vi "Event Log Monitor.vi"(8 "error in":errorcluster) -> (0 "error out":errorcluster, 3 "Log File Refnum":refnum<file>)   [LabVIEW 2019]
doc: "Does 2 Functions\n\n1. Creates log file name with date/time stamp upon first run\n2. Monitors log file size and closes current file and creates a new one when size limit is reached."
uses:
  Globals and Definitions/Initialization Globals.vi
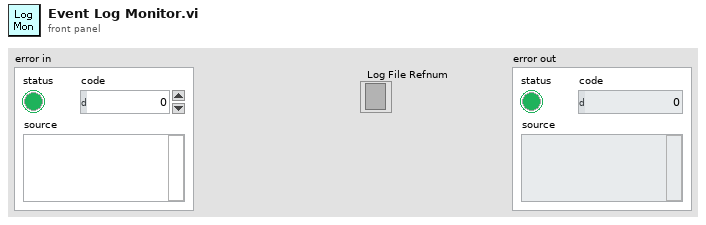
[diagram p1: front panel]
types:
  T1 = enum16{"open", "replace", "create", "open or create", "replace or create", "replace or create with confirmation"}
  T2 = typedef "LVDateTimeRec.ctl" = cluster{"fractional second":dbl, "second":i32, "minute":i32, "hour":i32, "day of month":i32, "month":i32, "year":i32, "day of week":i32, "day of year":i32, "DST":i32}
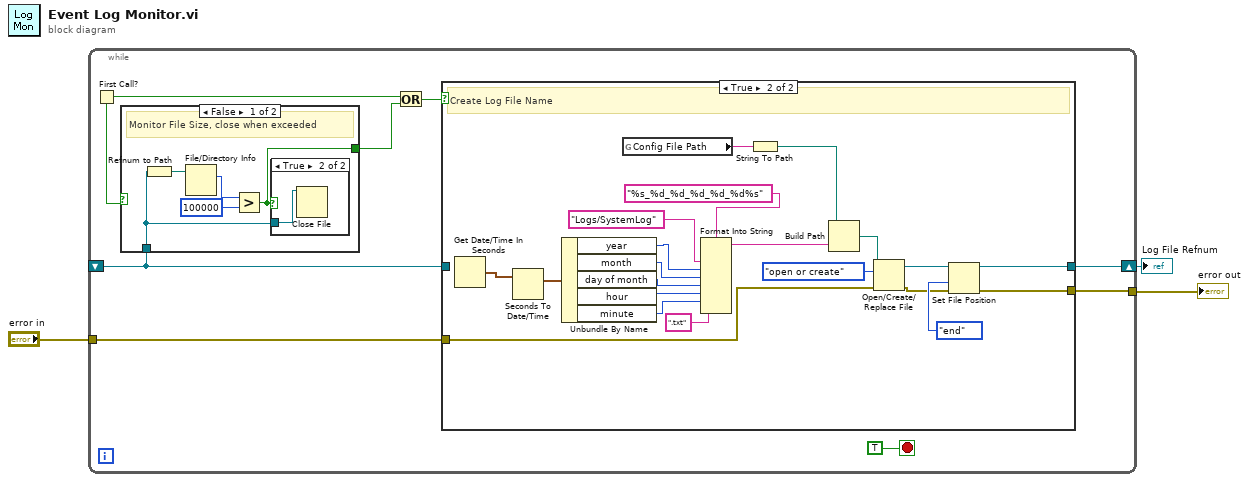
[diagram p0: block diagram]
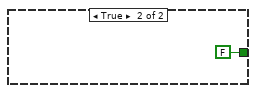
[diagram p3: hidden frame]
diagram:
  n1 = while {
    tunnel: "error in" -> [w11]
    tunnel: [w10] -> w2
    shift-right: [w8] -> w1
    shift-left: _ -> [w7]
    stop <- TRUE stop-if-true
    n2 = First Call?() -> (First Call?: T/F=w5:bool)
    n3 = case shown="False" w5 {
      tunnel: w7 -> [w13 _]
      tunnel: [w12 FALSE] -> w4
      frame False {
        # "Monitor File Size, close when exceeded"
        n4 = Refnum to Path(1:w13) -> (0:w16:path)
        n5 = File/Directory Info(path=w16) -> (size=w15:i64)  [unwired: 1 in, 6 out]
        n6 = Greater?(x=w15, y=i64 100000) -> (0:w12:bool)
        n7 = case shown="True" w12 {
          tunnel: w13 -> [_ w17]
          frame False {
          }
          frame True {
            n8 = Close File(refnum=w17) -> ()  [unwired: 1 in, 2 out]
          }
        }
      }
      frame True {
      }
    }
    n9 = Or(x=w5, y=w4) -> (x .or. y?=w6:bool)
    n10 = case shown="True" w6 {
      tunnel: w11 -> [w19 w27]
      tunnel: [w19 w25] -> w10
      tunnel: [w20 w22] -> w8
      tunnel: w7 -> [w20 _]
      frame False {
      }
      frame True {
        # "Create Log File Name"
        n11 = Get Date/Time In Seconds() -> (seconds since 1Jan1904=w28:timestamp)
        n12 = Seconds To Date/Time(time stamp (now)=w28) -> (date time rec=w41:T2)  [unwired: 1 in]
        n13 = Unbundle By Name(w41) -> ("year"=w34:i32, "month"=w33:i32, "day of month"=w32:i32, "hour"=w31:i32, "minute"=w30:i32)
        n14 = global read "Initialization Globals.vi" "Config File Path"() -> (w24:string)
        n15 = Format Into String(format string="%s_%d_%d_%d_%d_%d%s", "Logs/SystemLog" ("name or relative path"), w34, w33, w32, w31, w30, ".txt" ("name or relative path")) -> (resulting string=w29:string)  [unwired: 2 in, 1 out]
        n16 = String To Path(string=w24) -> (path=w23:path)
        n17 = Build Path(base path=w23, name or relative path=w29) -> (appended path=w35:path)
        n18 = Open/Create/Replace File(file path (use dialog)=w35, error in=w27, operation (0:open)=T1."open or create") -> (refnum out=w21:refnum<file>, error out=w26:errorcluster)  [unwired: 3 in, 1 out]
        n19 = Set File Position(refnum=w21, from (0:start)=enum16{"start", "end", "current"}."end", error in=w26) -> (refnum out=w22:refnum<file>, error out=w25:errorcluster)  [unwired: 1 in]
      }
    }
  }
  "error out" <- w2
  "Log File Refnum" <- w1
